vi "String to Build Item.vi"(7 "Package Folder":path, 11 "String":string) -> (3 "Build Item":T1)   [LabVIEW 2020, in "neg-pkg.lvlib" / "Package.lvclass"]
uses:
  Package.lvclass
  Build Item.ctl
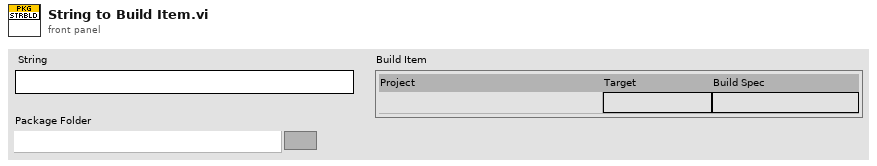
[diagram p1: front panel]
types:
  T1 = typedef "neg-pkg.lvlib/Package.lvclass/Build Item.ctl" = cluster{"Project":path, "Target":string, "Build Spec":string}
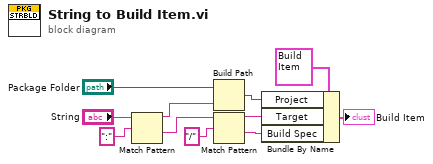
[diagram p0: block diagram]
diagram:
  n1 = Match Pattern(string="String", regular expression=":") -> (before substring=w6:string, after substring=w8:string)  [unwired: 1 in, 2 out]
  n2 = Build Path(base path="Package Folder", name or relative path=w6) -> (appended path=w3:path)
  n3 = Match Pattern(string=w8, regular expression="/") -> (before substring=w2:string, after substring=w1:string)  [unwired: 1 in, 2 out]
  n4 = Bundle By Name(cluster=T1 {"Project"=path "C:/dev/LabVIEW/neg-pkg/neg-pkg.lvproj", "Target"="My Computer", "Build Spec"="PPL"} ("Build Item"), "Project"=w3, "Target"=w2, "Build Spec"=w1) -> (→"Build Item":T1)
